vi "Read and Calc Digital.vi"() -> ()   [LabVIEW 2013]
panel:
  in  "АВП":bool=TRUE
  in  "Выбор предела":T1(ring)
  in  "Вариант":T2(ring)
  # "Обработка показаний цифрового вольтметра"
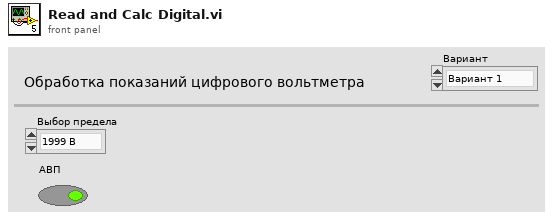
[diagram p1: front panel]
types:
  T1 = enum16{"1999 В", "199,9 В", "19,99 В", "1,999 В"}
  T2 = enum16{"Вариант 1", "Вариант 2", "Вариант 3", "Вариант 4", "Вариант 5", "Вариант 6", "Вариант 7", "Вариант 8", "Вариант 9", "Вариант 10", "Вариант 11", "Вариант 12"}
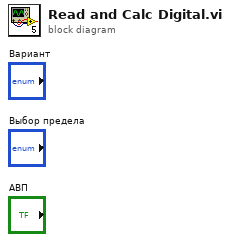
[diagram p0: block diagram]
diagram:
